vi "go_to_field.vi"(8 "Max Rates":dbl[][](array[numeric]), 9 "Timestep":dbl, 10 "Sweep To":dbl, 11 "VISA In":refnum<visa-resource-name>) -> (0 "B-Field":dbl, 3 "VISA Out":refnum<visa-resource-name>)   [LabVIEW 2016]
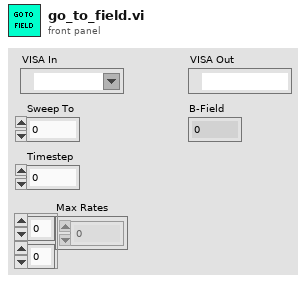
[diagram p1: front panel]
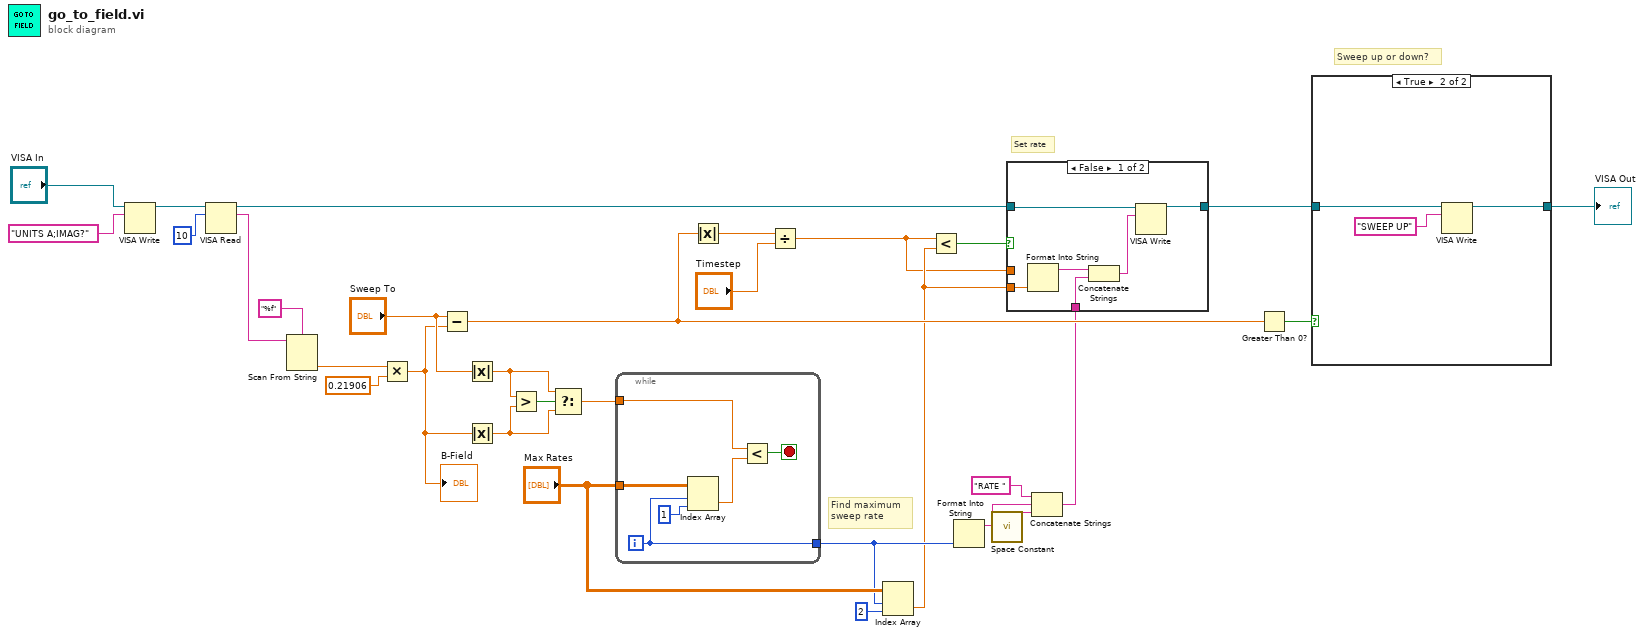
[diagram p0: block diagram]
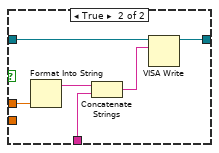
[diagram p2: hidden frame]
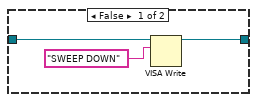
[diagram p3: hidden frame]
diagram:
  # "Set rate"
  # "Find maximum\nsweep rate"
  # "Sweep up or down?"
  n1 = VISA Write(VISA resource name="VISA In", write buffer="UNITS A;IMAG?") -> (VISA resource name out=w31:refnum<visa-resource-name>)  [unwired: 1 in, 2 out]
  n2 = VISA Read(VISA resource name=w31, byte count=u32 10) -> (VISA resource name out=w11:refnum<visa-resource-name>, read buffer=w27:string)  [unwired: 1 in, 2 out]
  n3 = Scan From String(format string="%f", input string=w27) -> (output 1=w24:dbl)  [unwired: 3 in, 3 out]
  n4 = Multiply(x=w24, y=0.21906) -> (x*y=w18:dbl)
  "B-Field" <- w18
  n5 = Subtract(x="Sweep To", y=w18) -> (x-y=w23:dbl)
  n6 = Absolute Value(x="Sweep To") -> (abs(x)=w16:dbl)
  n7 = Absolute Value(x=w18) -> (abs(x)=w17:dbl)
  n8 = Greater?(x=w16, y=w17) -> (0:w19:bool)
  n9 = Select(t=w16, s=w19, f=w17) -> (s? t:f=w15:dbl)
  n10 = while {
    tunnel: "Max Rates" -> [w37]
    tunnel: w15 -> [w35]
    tunnel: [w32] -> w10
    i -> [w32]
    stop <- w33 stop-if-true
    n11 = Index Array(array=w37, index (row)=w32, index (col)=1 ("disabled index (col)")) -> (element=w34:dbl)
    n12 = Less?(x=w35, y=w34) -> (x < y?=w33:bool)
  }
  n13 = Absolute Value(x=w23) -> (abs(x)=w22:dbl)
  n14 = Divide(x=w22, y="Timestep") -> (x/y=w5:dbl)
  n15 = Index Array(array="Max Rates", index (row)=w10, index (col)=2 ("disabled index (col)")) -> (element=w7:dbl)
  n16 = Less?(x=w5, y=w7) -> (x < y?=w13:bool)
  n17 = Format Into String(w10) -> (resulting string=w8:string)  [unwired: 3 in, 1 out]
  n18 = call <vilib>:"Space Constant.vi"() -> ("String"=w3:string)
  n19 = Concatenate Strings("RATE " ("string"), w8, w3) -> (w6:string)
  n20 = case shown="False" w13 {
    tunnel: [w43 w49] -> w12
    tunnel: w11 -> [w42 w48]
    tunnel: w7 -> [w41 _]
    tunnel: w6 -> [w39 w46]
    tunnel: w5 -> [_ w45]
    frame False {
      n21 = Format Into String(w41) -> (resulting string=w40:string)  [unwired: 3 in, 1 out]
      n22 = Concatenate Strings(w40, w39) -> (w38:string)
      n23 = VISA Write(VISA resource name=w42, write buffer=w38) -> (VISA resource name out=w43:refnum<visa-resource-name>)  [unwired: 1 in, 2 out]
    }
    frame True {
      n24 = Format Into String(w45) -> (resulting string=w47:string)  [unwired: 3 in, 1 out]
      n25 = Concatenate Strings(w47, w46) -> (w44:string)
      n26 = VISA Write(VISA resource name=w48, write buffer=w44) -> (VISA resource name out=w49:refnum<visa-resource-name>)  [unwired: 1 in, 2 out]
    }
  }
  n27 = Greater Than 0?(x=w23) -> (x > 0?=w29:bool)
  n28 = case shown="True" w29 {
    tunnel: w12 -> [w51 w54]
    tunnel: [w50 w53] -> w2
    frame False {
      n29 = VISA Write(VISA resource name=w51, write buffer="SWEEP DOWN") -> (VISA resource name out=w50:refnum<visa-resource-name>)  [unwired: 1 in, 2 out]
    }
    frame True {
      n30 = VISA Write(VISA resource name=w54, write buffer="SWEEP UP") -> (VISA resource name out=w53:refnum<visa-resource-name>)  [unwired: 1 in, 2 out]
    }
  }
  "VISA Out" <- w2
